vi "encodeStream.vi"(8 "error in (no error)":errorcluster, 11 "tBSON_I64 in":refnum<class "tBSON_I64.lvclass">) -> (0 "error out":errorcluster, 2 "Byte Array":u8[](array[numeric]), 3 "tBSON_I64 out":refnum<class "tBSON_I64.lvclass">)   [LabVIEW 2013, in "BSON.lvlib" / "tBSON_I64.lvclass"]
uses:
  tBSON_I64.lvclass
  tBSONElement/tBSONElement.lvclass
  getValue.vi
  BSON.lvlib
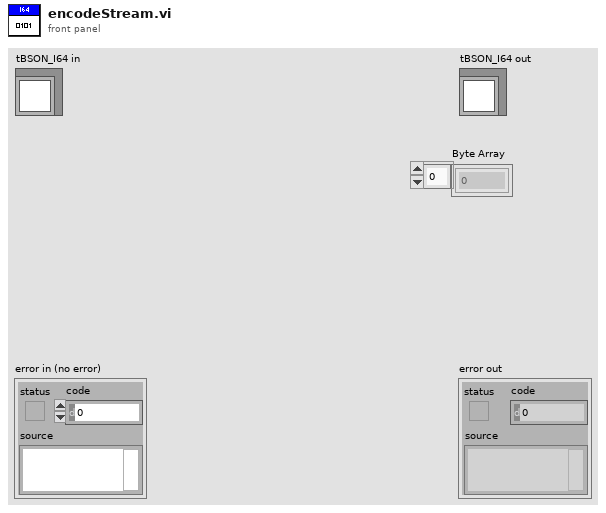
[diagram p1: front panel]
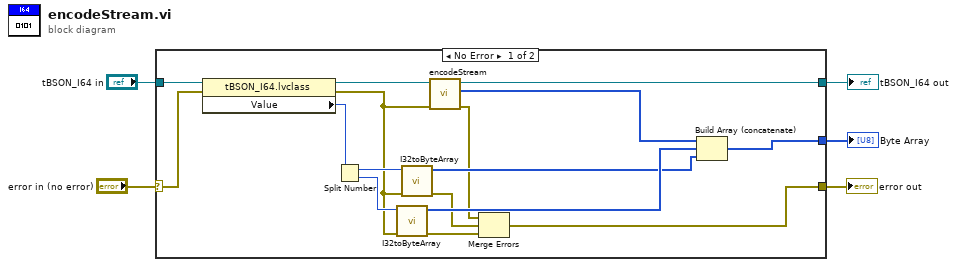
[diagram p0: block diagram]
diagram:
  n1 = case shown="No Error" "error in (no error)" {
    selector: "error in (no error)" -> [w20 w22]
    tunnel: "tBSON_I64 in" -> [w21 w23]
    tunnel: [w6 w23] -> w4
    tunnel: [w16 w22] -> w1
    tunnel: [w19 _] -> w3
    frame No Error {
      n2 = property class="tBSON_I64.lvclass"(reference=w21, error in=w20) -> (reference out=w10:refnum<class "tBSON_I64.lvclass">, error out=w9:errorcluster, "Value"=w15:i64)
      n3 = Split Number(x=w15) -> (hi(x)=w13:u32, lo(x)=w14:u32)
      n4 = call "I32toByteArray.vi"("error in (no error)"=w9, "I32"=w14) -> ("error out"=w17:errorcluster, "LittleEndianByteArray"=w18:u8[])  [unwired: 8 in]
      n5 = call "I32toByteArray.vi"("error in (no error)"=w9, "I32"=w13) -> ("error out"=w12:errorcluster, "LittleEndianByteArray"=w11:u8[])  [unwired: 8 in]
      n6 = call-parent "encodeStream.vi"("error in (no error)"=w9, "tBSONElement in"=w10) -> ("error out"=w8:errorcluster, "Byte Array"=w7:u8[], "tBSONElement out"=w6:refnum<class "tBSON_I64.lvclass">)  [unwired: 7 in]
      n7 = Merge Errors(w8, w12, w17) -> (w16:errorcluster)
      n8 = Build Array (concatenate)(w7, w18, w11) -> (w19:u8[])
    }
    frame Error {
    }
  }
  "error out" <- w1
  "tBSON_I64 out" <- w4
  "Byte Array" <- w3
